vi "Node.vi"() -> ()   [LabVIEW 2016]
uses:
  <vilib>/Utility/error.llb/DialogType.ctl
  <vilib>/pximc/Initialize Writer Session (DBL).vi
  <vilib>/pximc/Initialize Reader Session (DBL).vi
  <vilib>/pximc/Connect (DBL).vi
  <vilib>/pximc/Acquire Write Region (DBL).vi
  <vilib>/pximc/Acquire Read Region (DBL).vi
  <vilib>/pximc/nipximc.lvlib
  <resource>/objmgr/pximc.rc
panel:
  out "session out 4":refnum<k21>="PXIMC2::1223"
  out "session out 3":refnum<k21>="PXIMC2::1226"
  out "session out 2":refnum<k21>="PXIMC2::1225"
  out "session out":refnum<k21>="PXIMC2::1224"
  out "Writer Node 2":T1(graph)
  out "Writer Node 1":T1(graph)
  out "Stopped?":bool
  in  "Stop Button":bool
  in  "#Writing Channels Slave 2":i32=100
  in  "#Reading Channels Slave 2":i32=200
  out "Reader Node 2":T1(graph)
  in  "#Reading Channels Slave 1":i32=200
  in  "#Writing Channels Slave 1":i32=100
  out "Reader Node 1":T1(graph)
  in  "Node 1 Reader Connection ID":u16=4
  in  "Reader Interface Node 2":tag="PXIMC2" caption="interface"
  in  "Node 2 Writer Connection ID":u16=3
  in  "Writer Interface Node 2":tag="PXIMC2" caption="interface"
  in  "Node 1 Writer Connection ID":u16=1
  in  "Node 1 Writer Interface":tag="PXIMC2" caption="interface"
  in  "Node 1 Reader Interface":tag="PXIMC2" caption="interface"
  in  "Buffer Size":u64=250000 caption="buffer size"
  in  "Connection Timeout (s)":dbl=60.0 caption="timeout in seconds (-1)"
  in  "Node 1 Reader Connection ID":u16=2
  # "Node 1"
  # "Node 2"
  # "Node 2 => Node 1"
  # "Node 1 => Node 2"
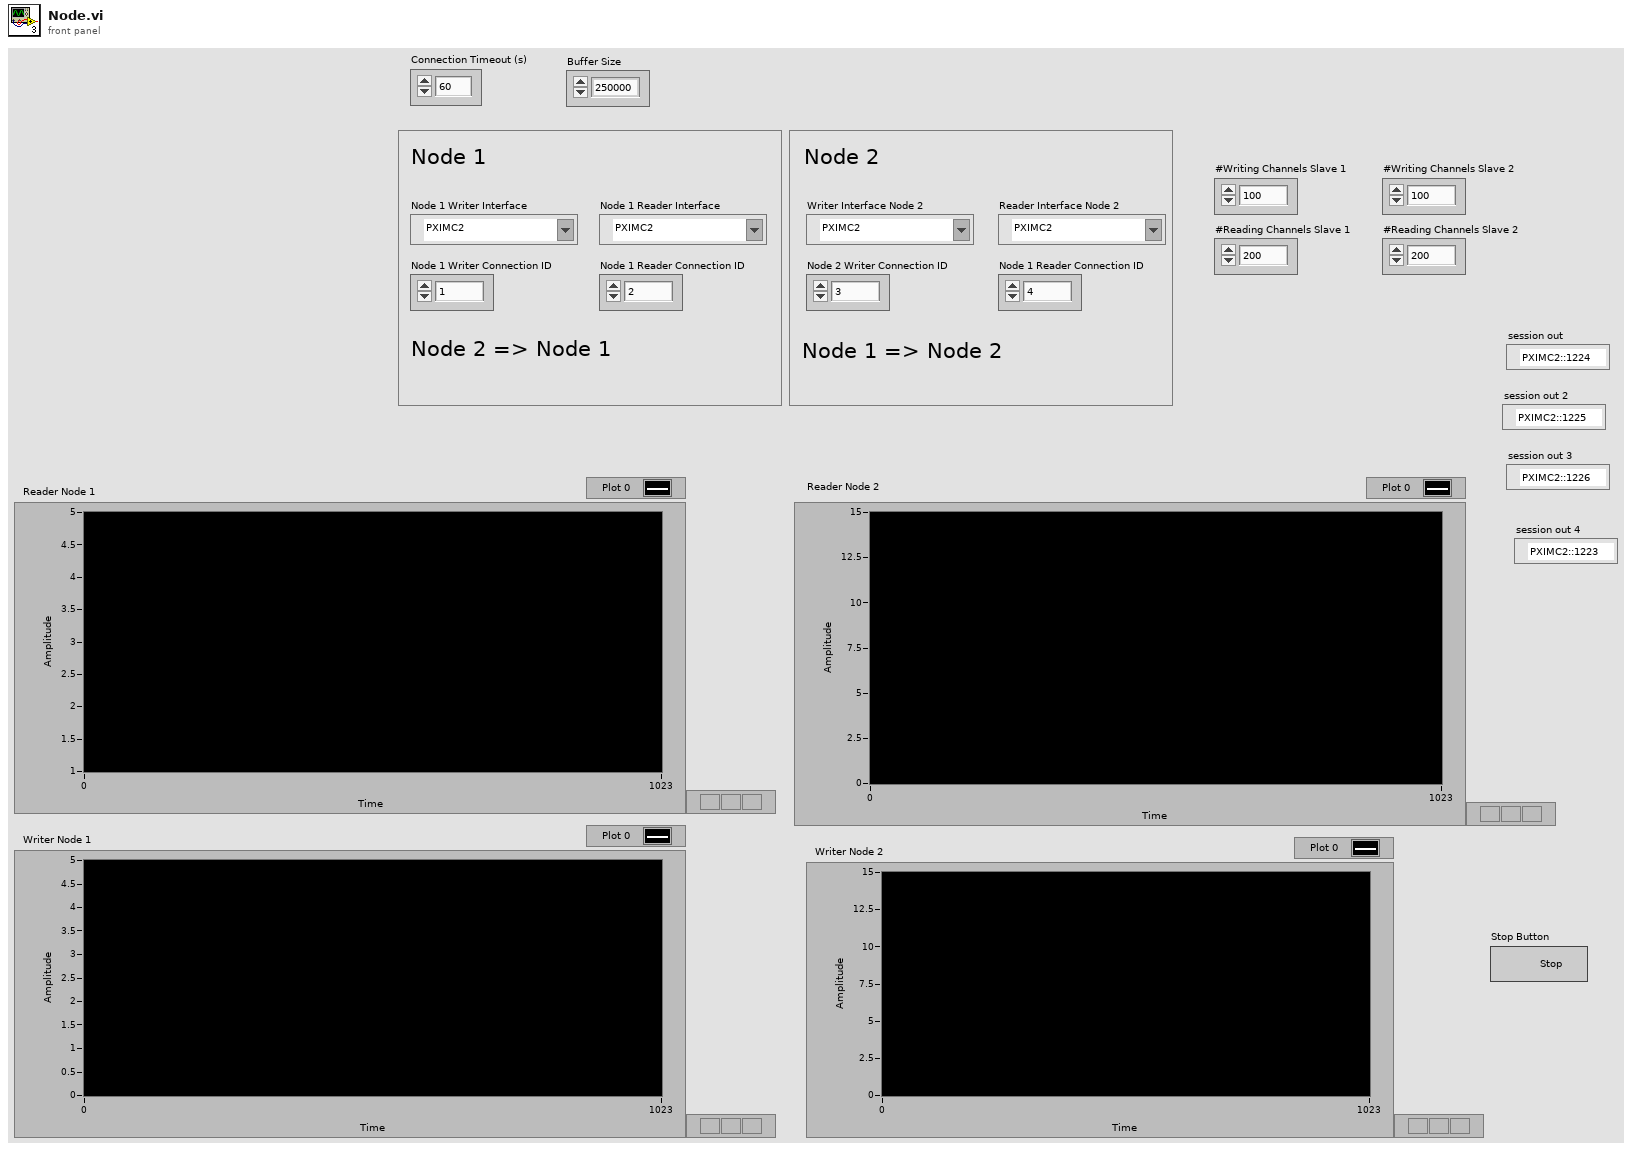
[diagram p1: front panel]
types:
  T1 = cluster{"[0]":dbl, "[1]":dbl, "[2]":dbl, "[3]":dbl, "[4]":dbl, "[5]":dbl, "[6]":dbl, "[7]":dbl, "[8]":dbl, "[9]":dbl, "[10]":dbl, "[11]":dbl, "[12]":dbl, "[13]":dbl, "[14]":dbl, "[15]":dbl, "[16]":dbl, "[17]":dbl, "[18]":dbl, "[19]":dbl}
  T2 = typedef "DialogType.ctl" = u16
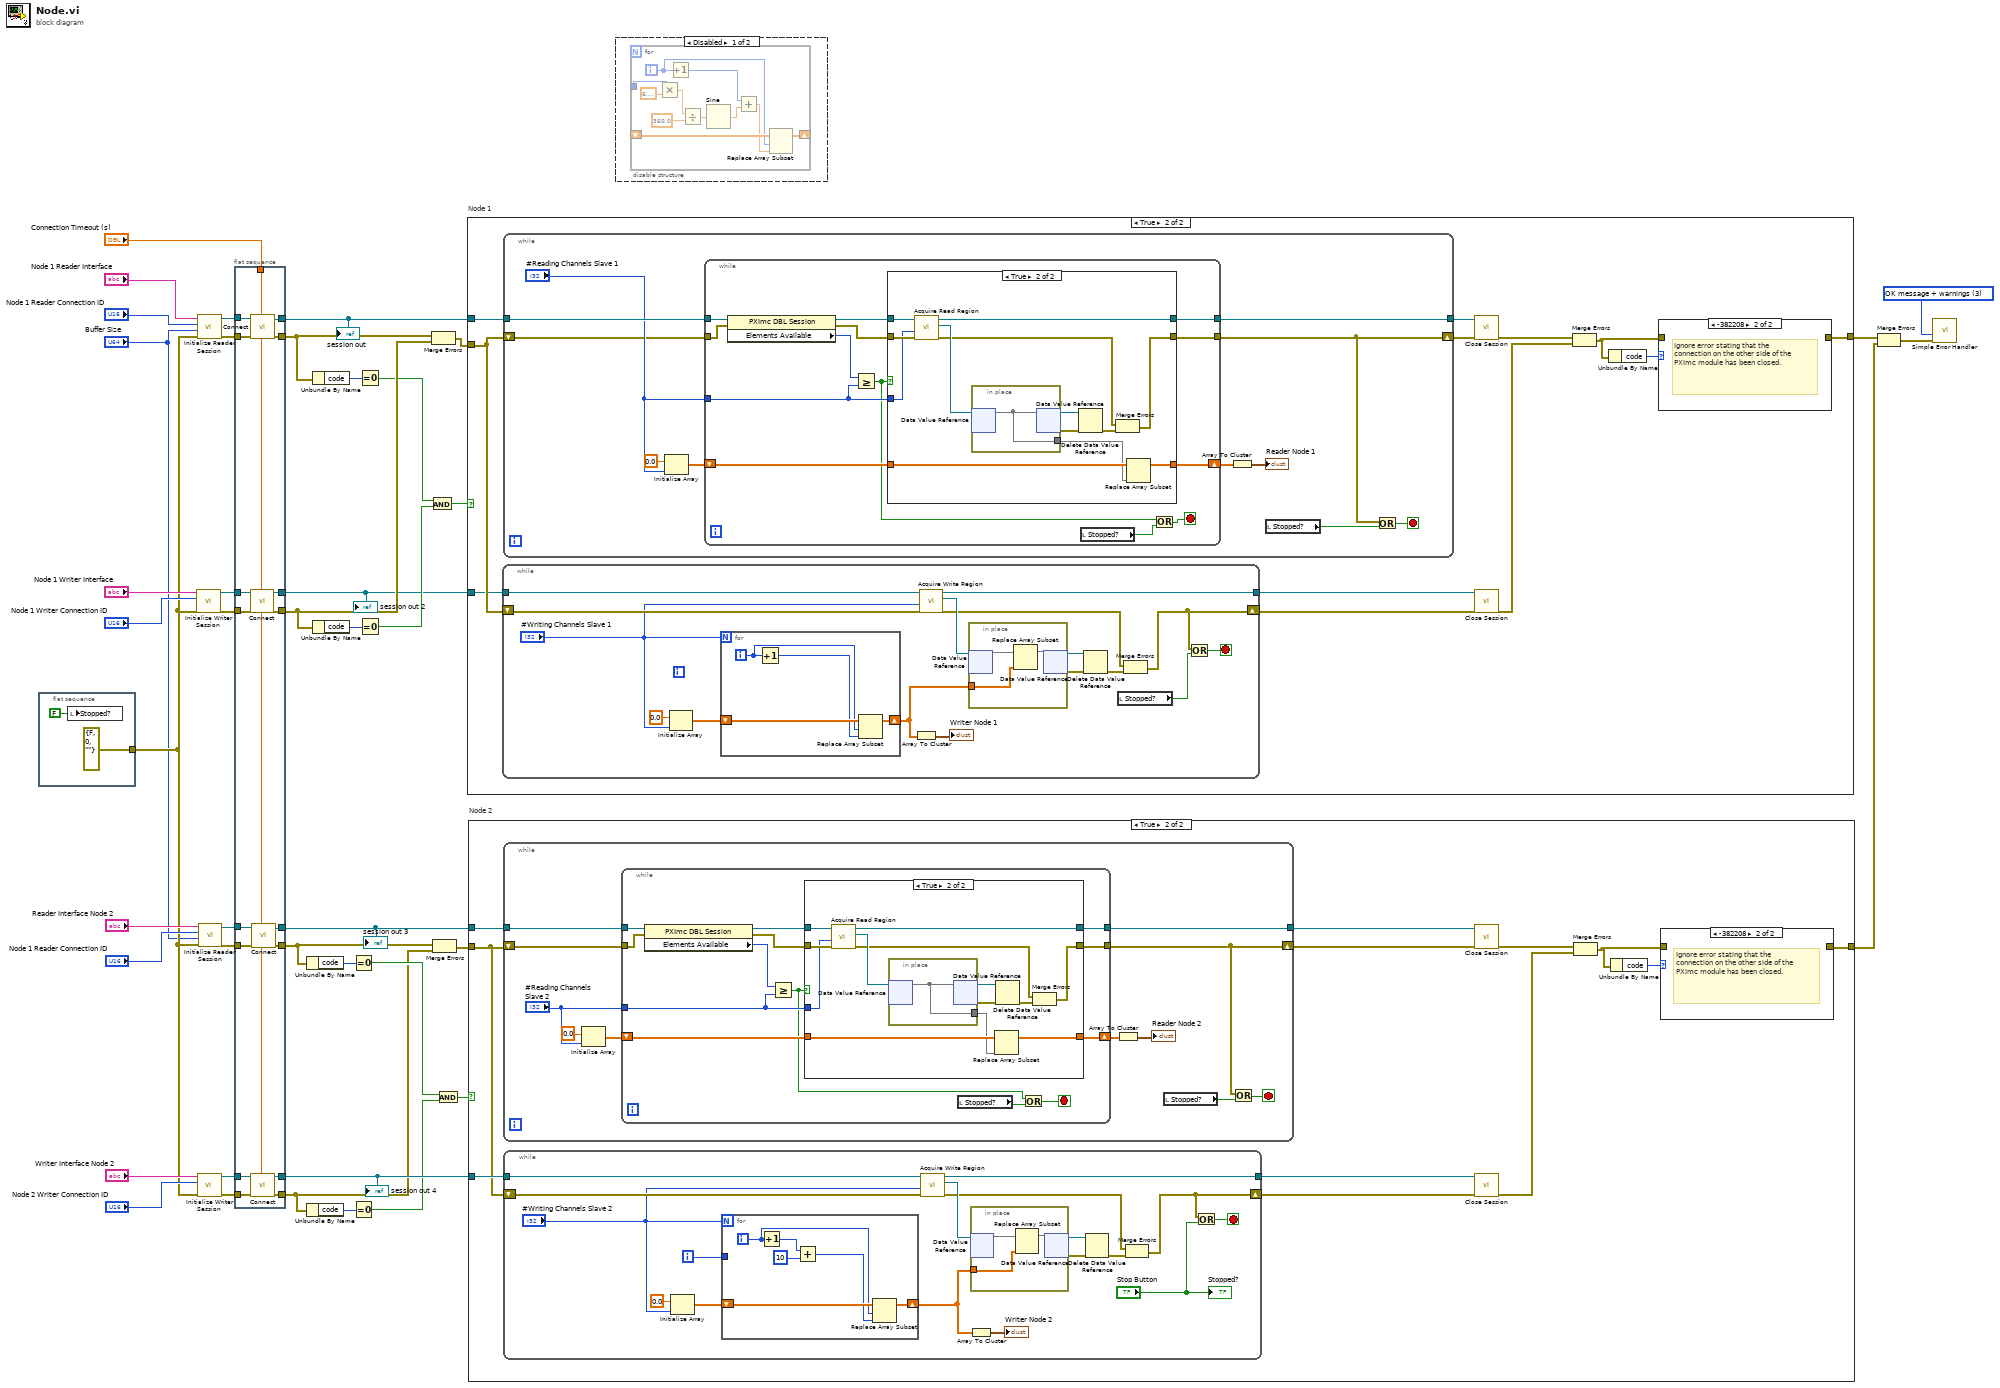
[diagram p0: block diagram]
diagram:
  w37 = T2 3 items=["no dialog", "OK message", "continue or stop message", "OK message + warnings", "continue/stop + warnings"] ("type of dialog (OK msg:1)")
  n1 = flat-sequence {
    tunnel: [errorcluster {"status"=FALSE, "code"=0, "source"=""} ("error constant")] -> w15
    frame #0 {
      n2 = local write "Stopped?"(FALSE ("Stopped?")) -> ()
    }
  }
  n3 = call-poly <vilib>:"Initialize Writer Session.vi"("error in (no error)"=w15, "connection id (1)"="Node 1 Writer Connection ID", "interface"="Node 1 Writer Interface") -> ("error out"=w35:errorcluster, "session out"=w34:refnum<k21>)  [unwired: 7 in]
  n4 = call-poly <vilib>:"Initialize Reader Session.vi"("error in (no error)"=w15, "buffer size"="Buffer Size", "writer's connection id (1)"="Node 1 Reader Connection ID", "interface"="Node 1 Reader Interface") -> ("error out"=w41:errorcluster, "session out"=w42:refnum<k21>)  [unwired: 6 in]
  n5 = call-poly <vilib>:"Initialize Writer Session.vi"("error in (no error)"=w15, "connection id (1)"="Node 2 Writer Connection ID", "interface"="Writer Interface Node 2") -> ("error out"=w22:errorcluster, "session out"=w23:refnum<k21>)  [unwired: 7 in]
  n6 = call-poly <vilib>:"Initialize Reader Session.vi"("error in (no error)"=w15, "buffer size"="Buffer Size", "writer's connection id (1)"="Node 1 Reader Connection ID", "interface"="Reader Interface Node 2") -> ("error out"=w18:errorcluster, "session out"=w17:refnum<k21>)  [unwired: 6 in]
  n7 = flat-sequence {
    tunnel: w42 -> [w62]
    tunnel: w41 -> [w61]
    tunnel: [w60] -> w40
    tunnel: w35 -> [w59]
    tunnel: w34 -> [w58]
    tunnel: [w57] -> w29
    tunnel: [w56] -> w28
    tunnel: "Connection Timeout (s)" -> [w46]
    tunnel: [w55] -> w26
    tunnel: [w54] -> w11
    tunnel: [w53] -> w3
    tunnel: [w52] -> w4
    tunnel: w23 -> [w51]
    tunnel: w22 -> [w50]
    tunnel: [w49] -> w12
    tunnel: w18 -> [w48]
    tunnel: w17 -> [w47]
    frame #0 {
      n8 = call-poly <vilib>:"Connect.vi"("timeout in seconds (-1)"=w46, "error in (no error)"=w59, "session in"=w58) -> ("error out"=w56:errorcluster, "session out"=w55:refnum<k21>)  [unwired: 7 in]
      n9 = call-poly <vilib>:"Connect.vi"("timeout in seconds (-1)"=w46, "error in (no error)"=w61, "session in"=w62) -> ("error out"=w57:errorcluster, "session out"=w60:refnum<k21>)  [unwired: 7 in]
      n10 = call-poly <vilib>:"Connect.vi"("timeout in seconds (-1)"=w46, "error in (no error)"=w50, "session in"=w51) -> ("error out"=w53:errorcluster, "session out"=w54:refnum<k21>)  [unwired: 7 in]
      n11 = call-poly <vilib>:"Connect.vi"("timeout in seconds (-1)"=w46, "error in (no error)"=w48, "session in"=w47) -> ("error out"=w52:errorcluster, "session out"=w49:refnum<k21>)  [unwired: 7 in]
    }
  }
  n12 = Unbundle By Name(w4) -> ("code"=w20:i32)
  n13 = Unbundle By Name(w3) -> ("code"=w25:i32)
  n14 = Unbundle By Name(w29) -> ("code"=w38:i32)
  n15 = Unbundle By Name(w28) -> ("code"=w32:i32)
  n16 = Equal To 0?(x=w20) -> (x = 0?=w6:bool)
  n17 = Equal To 0?(x=w25) -> (x = 0?=w5:bool)
  n18 = Equal To 0?(x=w38) -> (x = 0?=w13:bool)
  n19 = Equal To 0?(x=w32) -> (x = 0?=w31:bool)
  n20 = And(x=w13, y=w31) -> (x .and. y?=w8:bool)
  n21 = Merge Errors(w29, w28) -> (w30:errorcluster)
  n22 = Merge Errors(w4, w3) -> (w2:errorcluster)
  n23 = And(x=w6, y=w5) -> (x .and. y?=w7:bool)
  n24 = case "Node 1" shown="True" w8 {
    tunnel: w40 -> [_ w75]
    tunnel: w30 -> [w63 w74]
    tunnel: w26 -> [_ w73]
    tunnel: [w63 w72] -> w10
    frame False {
    }
    frame True {
      n25 = while {
        tunnel: w73 -> [w84]
        tunnel: [w83] -> w69
        shift-right: [w80] -> w67
        shift-left: w74 -> [w82]
        stop <- w79 stop-if-true
        n26 = Initialize Array(0.0 ("element"), "#Writing Channels Slave 1") -> (w91:dbl[])
        n27 = for {
          N: "#Writing Channels Slave 1" -> [_]
          shift-right: [w97] -> w76
          shift-left: w91 -> [w98]
          i -> [w96]
          n28 = Increment(x=w96) -> (x+1=w95:i32)
          n29 = Replace Array Subset(array=w98, new element=w95, index=w96) -> (w97:dbl[])
        }
        n30 = Array To Cluster(array=w76) -> (cluster=→"Writer Node 1":T1)
        n31 = call-poly <vilib>:"Acquire Write Region.vi"("error in (no error)"=w82, "number of elements"="#Writing Channels Slave 1", "session in"=w84) -> ("error out"=w85:errorcluster, "write region reference"=w86:refnum<data-value>, "session out"=w83:refnum<k21>)  [unwired: 5 in, 1 out]
        n32 = in-place {
          in-place-border: w76 -> [w92]
          n33 = in-place-dvr #1(w86) -> (w94:dbl[])  [unwired: 1 out]
          n34 = Replace Array Subset(array=w94, new element=w92) -> (w93:dbl[])  [unwired: 1 in]
          n35 = in-place-dvr #1(w93) -> (w87:refnum<data-value>, w89:errorcluster)
        }
        n36 = Delete Data Value Reference(data value reference=w87, error in=w89) -> (error out=w88:errorcluster)  [unwired: 1 out]
        n37 = local read "Stopped?"() -> (w78:bool)
        n38 = Merge Errors(w85, w88) -> (w80:errorcluster)
        n39 = Or(x=w80, y=w78) -> (x .or. y?=w79:bool)
      }
      n40 = while {
        tunnel: [w103] -> w70
        shift-right: [w102] -> w68
        shift-left: w74 -> [w100]
        tunnel: w75 -> [w107]
        stop <- w109 stop-if-true
        n41 = Initialize Array(0.0 ("element"), "#Reading Channels Slave 1") -> (w106:dbl[])
        n42 = while {
          tunnel: w107 -> [w121]
          tunnel: w100 -> [w118]
          tunnel: [w122] -> w102
          tunnel: "#Reading Channels Slave 1" -> [w114]
          shift-right: [w115] -> w101
          shift-left: w106 -> [w116]
          tunnel: [w113] -> w103
          stop <- w110 stop-if-true
          n43 = property class="PXImc DBL Session"(reference=w121, error in=w118) -> (reference out=w119:refnum<k21>, error out=w117:errorcluster, "Elements Available"=w120:u64)
          n44 = Greater Or Equal?(x=w120, y=w114) -> (x >= y?=w112:bool)
          n45 = case shown="True" w112 {
            tunnel: w117 -> [w125 w137]
            tunnel: [w125 w131] -> w122
            tunnel: w119 -> [w123 w136]
            tunnel: w116 -> [w124 w130]
            tunnel: [w124 w128] -> w115
            tunnel: w114 -> [_ w127]
            tunnel: [w123 w126] -> w113
            frame False {
            }
            frame True {
              n46 = call-poly <vilib>:"Acquire Read Region.vi"("error in (no error)"=w137, "number of elements"=w127, "session in"=w136) -> ("error out"=w132:errorcluster, "read region reference"=w138:refnum<data-value>, "session out"=w126:refnum<k21>)  [unwired: 5 in, 1 out]
              n47 = in-place {
                in-place-border: [w139] -> w129
                n48 = in-place-dvr #2(w138) -> (w139:dbl[])  [unwired: 1 out]
                n49 = in-place-dvr #2(w139) -> (w135:refnum<data-value>, w134:errorcluster)
              }
              n50 = Delete Data Value Reference(data value reference=w135, error in=w134) -> (error out=w133:errorcluster)  [unwired: 1 out]
              n51 = Merge Errors(w132, w133) -> (w131:errorcluster)
              n52 = Replace Array Subset(array=w130, new element=w129) -> (w128:dbl[])  [unwired: 1 in]
            }
          }
          n53 = local read "Stopped?"() -> (w111:bool)
          n54 = Or(x=w112, y=w111) -> (x .or. y?=w110:bool)
        }
        n55 = Array To Cluster(array=w101) -> (cluster=→"Reader Node 1":T1)
        n56 = local read "Stopped?"() -> (w99:bool)
        n57 = Or(x=w102, y=w99) -> (x .or. y?=w109:bool)
      }
      n58 = call <vilib>:"Close Session.vi"("error in (no error)"=w68, "session in"=w70) -> ("error out"=w66:errorcluster)  [unwired: 9 in]
      n59 = call <vilib>:"Close Session.vi"("error in (no error)"=w67, "session in"=w69) -> ("error out"=w65:errorcluster)  [unwired: 9 in]
      n60 = Merge Errors(w66, w65) -> (w64:errorcluster)
      n61 = Unbundle By Name(w64) -> ("code"=w71:i32)
      n62 = case shown="-382208" w71 {
        tunnel: w64 -> [w140 _]
        tunnel: [w140 _] -> w72
        frame 0, Default {
        }
        frame -382208 {
          # "Ignore error stating that the connection on the other side of the PXImc module has been closed."
        }
      }
    }
  }
  n63 = case "Node 2" shown="True" w7 {
    tunnel: w12 -> [_ w153]
    tunnel: w11 -> [_ w152]
    tunnel: w2 -> [w141 w143]
    tunnel: [w141 w142] -> w1
    frame False {
    }
    frame True {
      n64 = while {
        tunnel: [w185] -> w150
        shift-right: [w182] -> w149
        shift-left: w143 -> [w183]
        tunnel: w153 -> [w189]
        stop <- w191 stop-if-true
        n65 = Initialize Array(0.0 ("element"), "#Reading Channels Slave 2") -> (w188:dbl[])
        n66 = while {
          tunnel: w189 -> [w203]
          tunnel: w183 -> [w200]
          tunnel: [w204] -> w182
          tunnel: "#Reading Channels Slave 2" -> [w196]
          shift-right: [w197] -> w184
          shift-left: w188 -> [w198]
          tunnel: [w195] -> w185
          stop <- w192 stop-if-true
          n67 = property class="PXImc DBL Session"(reference=w203, error in=w200) -> (reference out=w201:refnum<k21>, error out=w199:errorcluster, "Elements Available"=w202:u64)
          n68 = Greater Or Equal?(x=w202, y=w196) -> (x >= y?=w193:bool)
          n69 = case shown="True" w193 {
            tunnel: w199 -> [w207 w219]
            tunnel: [w207 w213] -> w204
            tunnel: w201 -> [w205 w218]
            tunnel: w198 -> [w206 w212]
            tunnel: [w206 w210] -> w197
            tunnel: w196 -> [_ w209]
            tunnel: [w205 w208] -> w195
            frame False {
            }
            frame True {
              n70 = call-poly <vilib>:"Acquire Read Region.vi"("error in (no error)"=w219, "number of elements"=w209, "session in"=w218) -> ("error out"=w214:errorcluster, "read region reference"=w220:refnum<data-value>, "session out"=w208:refnum<k21>)  [unwired: 5 in, 1 out]
              n71 = in-place {
                in-place-border: [w221] -> w211
                n72 = in-place-dvr #3(w220) -> (w221:dbl[])  [unwired: 1 out]
                n73 = in-place-dvr #3(w221) -> (w217:refnum<data-value>, w216:errorcluster)
              }
              n74 = Replace Array Subset(array=w212, new element=w211) -> (w210:dbl[])  [unwired: 1 in]
              n75 = Delete Data Value Reference(data value reference=w217, error in=w216) -> (error out=w215:errorcluster)  [unwired: 1 out]
              n76 = Merge Errors(w214, w215) -> (w213:errorcluster)
            }
          }
          n77 = local read "Stopped?"() -> (w194:bool)
          n78 = Or(x=w193, y=w194) -> (x .or. y?=w192:bool)
        }
        n79 = Array To Cluster(array=w184) -> (cluster=→"Reader Node 2":T1)
        n80 = local read "Stopped?"() -> (w181:bool)
        n81 = Or(x=w182, y=w181) -> (x .or. y?=w191:bool)
      }
      n82 = while {
        tunnel: w152 -> [w164]
        tunnel: [w163] -> w151
        shift-right: [w160] -> w148
        shift-left: w143 -> [w162]
        i -> [w157]
        stop <- w159 stop-if-true
        n83 = Initialize Array(0.0 ("element"), "#Writing Channels Slave 2") -> (w171:dbl[])
        n84 = for {
          N: "#Writing Channels Slave 2" -> [_]
          tunnel: w157 -> [_]
          shift-right: [w179] -> w155
          shift-left: w171 -> [w180]
          i -> [w178]
          n85 = Increment(x=w178) -> (x+1=w177:i32)
          n86 = Add(x=w177, y=10) -> (x+y=w175:i32)
          n87 = Replace Array Subset(array=w180, new element=w175, index=w178) -> (w179:dbl[])
        }
        n88 = call-poly <vilib>:"Acquire Write Region.vi"("error in (no error)"=w162, "number of elements"="#Writing Channels Slave 2", "session in"=w164) -> ("error out"=w165:errorcluster, "write region reference"=w166:refnum<data-value>, "session out"=w163:refnum<k21>)  [unwired: 5 in, 1 out]
        n89 = Array To Cluster(array=w155) -> (cluster=→"Writer Node 2":T1)
        n90 = in-place {
          in-place-border: w155 -> [w172]
          n91 = in-place-dvr #4(w166) -> (w174:dbl[])  [unwired: 1 out]
          n92 = Replace Array Subset(array=w174, new element=w172) -> (w173:dbl[])  [unwired: 1 in]
          n93 = in-place-dvr #4(w173) -> (w167:refnum<data-value>, w169:errorcluster)
        }
        n94 = Delete Data Value Reference(data value reference=w167, error in=w169) -> (error out=w168:errorcluster)  [unwired: 1 out]
        n95 = Merge Errors(w165, w168) -> (w160:errorcluster)
        n96 = Or(x=w160, y="Stop Button") -> (x .or. y?=w159:bool)
        "Stopped?" <- "Stop Button"
      }
      n97 = call <vilib>:"Close Session.vi"("error in (no error)"=w149, "session in"=w150) -> ("error out"=w145:errorcluster)  [unwired: 9 in]
      n98 = call <vilib>:"Close Session.vi"("error in (no error)"=w148, "session in"=w151) -> ("error out"=w144:errorcluster)  [unwired: 9 in]
      n99 = Merge Errors(w145, w144) -> (w146:errorcluster)
      n100 = Unbundle By Name(w146) -> ("code"=w147:i32)
      n101 = case shown="-382208" w147 {
        tunnel: w146 -> [w154 _]
        tunnel: [w154 _] -> w142
        frame 0, Default {
        }
        frame -382208 {
          # "Ignore error stating that the connection on the other side of the PXImc module has been closed."
        }
      }
    }
  }
  n102 = disable-structure shown="Disabled" {
    frame Disabled {
      n103 = for {
        tunnel: _ -> [w229]
        shift-right: [w227] -> _
        shift-left: _ -> [w228]
        i -> [w226]
        n104 = Multiply(x=w229, y=6.283185307179586) -> (x*y=w231:dbl)
        n105 = Increment(x=w226) -> (x+1=w223:i32)
        n106 = Divide(x=w231, y=360.0) -> (x/y=w225:dbl)
        n107 = Sine(x=w225) -> (sin(x)=w224:dbl)
        n108 = Add(x=w223, y=w224) -> (x+y=w222:dbl)
        n109 = Replace Array Subset(array=w228, new element=w222, index=w226) -> (w227:dbl[])
      }
    }
    frame Enabled {
    }
  }
  n110 = Merge Errors(w10, w1) -> (w9:errorcluster)
  n111 = call <vilib>:"Simple Error Handler.vi"("type of dialog (OK msg:1)"=w37, "error in (no error)"=w9) -> ()  [unwired: 3 in, 5 out]
  "session out" <- w40
  "session out 2" <- w26
  "session out 3" <- w12
  "session out 4" <- w11
